vi "Auto Indexing Array.vi"() -> ()   [LabVIEW 2015]
uses:
  Title - Type Def.ctl
  Employee Record - Type Def.ctl
panel:
  out "Count":i32
  out "Employee Record Out":T1[](array[typedef]) {"Start Date" format="%<%x %.3X>T"}
  in  "Employee Record In":T1[](array[typedef]) {"Start Date" format="%<%x %.3X>T"}
  out "Manipulated Array (For Loop)":dbl[](array[numeric])
  out "Manipulated Array (Loopless)":dbl[](array[numeric])
  in  "Array in":dbl[](array[numeric])
  out "Array of random numbers":dbl[](array[numeric])
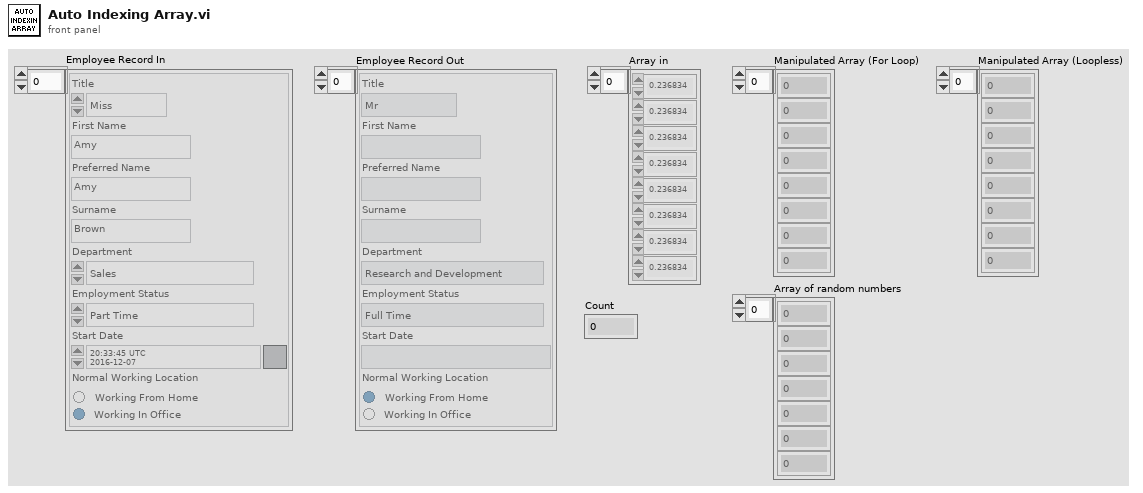
[diagram p1: front panel]
types:
  T1 = typedef "Employee Record - Type Def.ctl" = cluster{"Title":T2, "First Name":string, "Preferred Name":string, "Surname":string, "Department":enum16{"Research and Development", "Technical Support", "Sales", "Management", "Finance", "Other"}, "Employment Status":enum16{"Full Time", "Part Time", "No Longer Employed", "Probation", "Other"}, "Start Date":timestamp, "Normal Working Location":enum32{"Working From Home", "Working in Office"}}
  T2 = typedef "Title - Type Def.ctl" = enum16{"Mr", "Mrs", "Ms", "Mx", "Miss", "Sir", "Dame", "Other"}
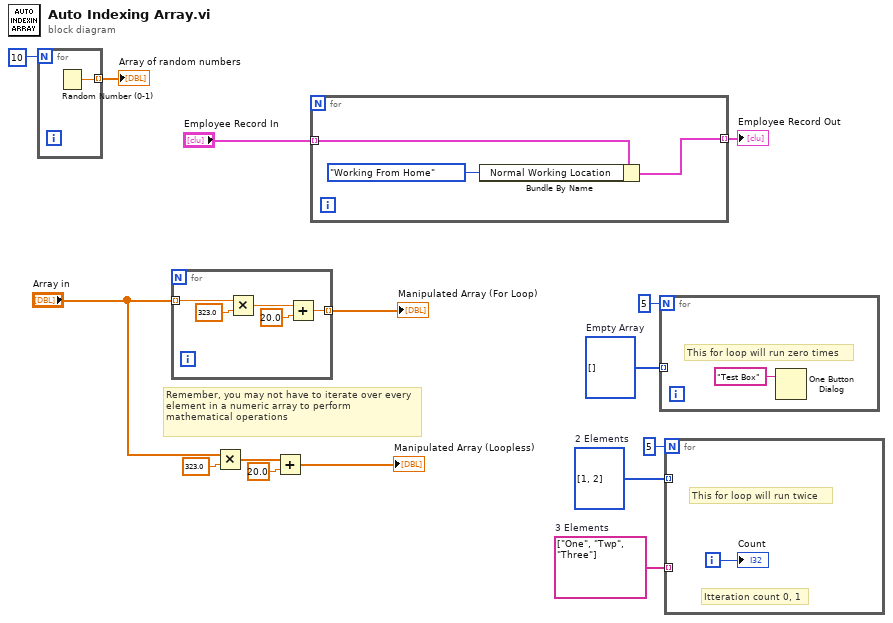
[diagram p0: block diagram]
diagram:
  w1 = string[] ["One", "Twp", "Three"]  # 3 Elements
  w3 = i32[] [1, 2]  # 2 Elements
  w4 = i32[] []  # Empty Array
  # "Remember, you may not have to iterate over every element in a numeric array to perform mathematical operations"
  n1 = for {
    N: 10 -> [_]
    tunnel: [w16] -> w15 mode=indexing
    n2 = Random Number (0-1)() -> (number: 0 to 1=w16:dbl)
  }
  "Array of random numbers" <- w15
  n3 = for {
    tunnel: "Array in" -> [w21] mode=indexing
    tunnel: [w17] -> w8 mode=indexing
    n4 = Multiply(x=w21, y=323.0) -> (x*y=w19:dbl)
    n5 = Add(x=w19, y=20.0) -> (x+y=w17:dbl)
  }
  "Manipulated Array (For Loop)" <- w8
  n6 = Multiply(x="Array in", y=323.0) -> (x*y=w12:dbl[])
  n7 = Add(x=w12, y=20.0) -> (x+y=→"Manipulated Array (Loopless)":dbl[])
  n8 = for {
    tunnel: "Employee Record In" -> [w24] mode=indexing
    tunnel: [w22] -> w6 mode=indexing
    n9 = Bundle By Name(cluster=w24, "Normal Working Location"=enum32{"Working From Home", "Working in Office"}."Working From Home") -> (w22:T1)
  }
  "Employee Record Out" <- w6
  n10 = for {
    N: 5 -> [_]
    tunnel: w4 -> [_] mode=indexing
    # "This for loop will run zero times"
    n11 = One Button Dialog(message="Test Box") -> ()  [unwired: 1 in, 1 out]
  }
  n12 = for {
    N: 5 -> [_]
    tunnel: w3 -> [_] mode=indexing
    tunnel: w1 -> [_] mode=indexing
    i -> [w26]
    # "Itteration count 0, 1"
    # "This for loop will run twice"
    "Count" <- w26
  }
